vi "Calculate Block Duration.vi"(8 "error in (no error)":errorcluster, 11 "DAQ Task in":refnum<class "DAQ Task.lvclass">) -> (0 "error out":errorcluster, 2 "Block Duration (ms)":i32, 3 "DAQ Task out":refnum<class "DAQ Task.lvclass">)   [LabVIEW 2018, in "Data Acquisition.lvlib" / "DAQ Task.lvclass"]
uses:
  DAQ Task.lvclass
  DAQ Task.lvclass/DAQ Task.ctl
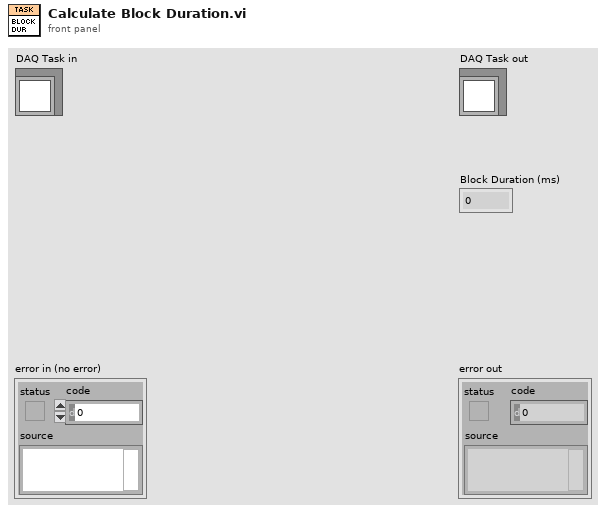
[diagram p1: front panel]
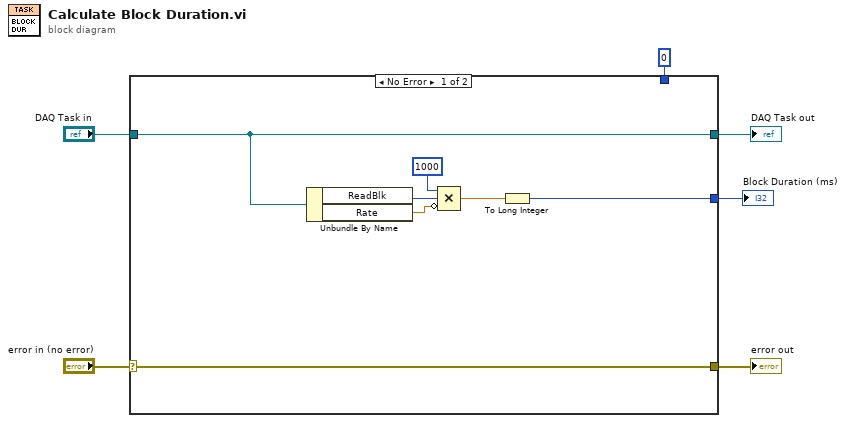
[diagram p0: block diagram]
diagram:
  n1 = case shown="No Error" "error in (no error)" {
    selector: "error in (no error)" -> [w13 w16]
    tunnel: [w13 w16] -> w5
    tunnel: [w12 w15] -> w3
    tunnel: "DAQ Task in" -> [w12 w15]
    tunnel: [w7 w14] -> w2
    tunnel: 0 -> [_ w14]
    frame No Error {
      n2 = Unbundle By Name(w12) -> ("ReadBlk"=w11:i32, "Rate"=w10:dbl)
      n3 = Compound Arithmetic op=MULTIPLY(1000 ("value"), w11, invert w10) -> (w8:dbl)
      n4 = To Long Integer(number=w8) -> (32bit integer=w7:i32)
    }
    frame Error {
    }
  }
  "error out" <- w5
  "DAQ Task out" <- w3
  "Block Duration (ms)" <- w2
